vi "HandshakeResponse.vi"(8 "error in (no error)":errorcluster, 10 "Sec-WebSocket-Key":string, 11 "WebSocket In":refnum<class "WebSocket.lvclass">) -> (0 "error out":errorcluster, 2 "Response Headers":string, 3 "WebSocket out":refnum<class "WebSocket.lvclass">)   [LabVIEW 2021, in "WebSockets.lvlib" / "WebSocket.lvclass"]
doc: "Creates the HTTP handshaking response.\nWebSockets 2.0.1.40\nSam Sharp - MediaMongrels Ltd\nCopyright (c) 2019, MediaMongrels Ltd"
uses:
  WebSocket.lvclass
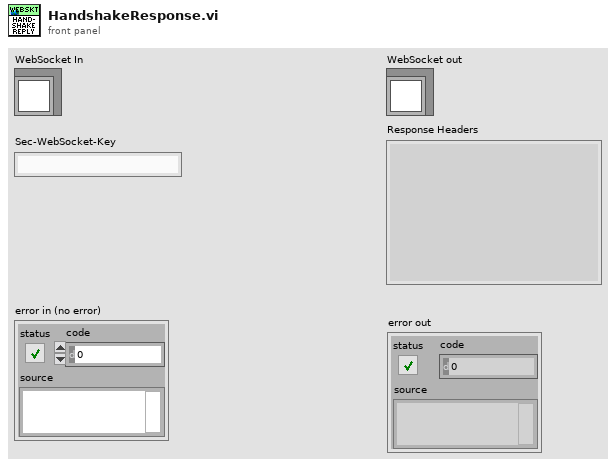
[diagram p1: front panel]
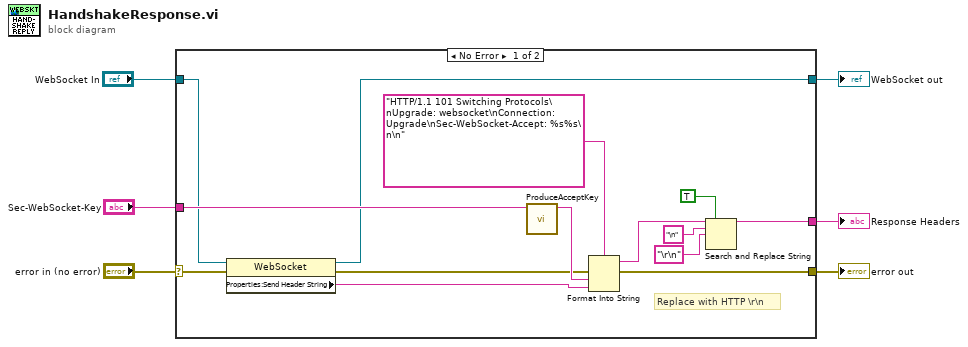
[diagram p0: block diagram]
diagram:
  n1 = case shown="No Error" "error in (no error)" {
    selector: "error in (no error)" -> [w17 w22]
    tunnel: "Sec-WebSocket-Key" -> [w20 _]
    tunnel: [w12 _] -> w5
    tunnel: [w18 w22] -> w3
    tunnel: "WebSocket In" -> [w10 w21]
    tunnel: [w7 w21] -> w1
    frame No Error {
      # "Replace with HTTP \\r\\n"
      n2 = property class="WebSocket"(reference=w10, error in=w17) -> (reference out=w7:refnum<class "WebSocket.lvclass">, error out=w11:errorcluster, "Properties:Send Header String"=w9:string)
      n3 = call "ProduceAcceptKey.vi"("Sec-WebSocket-Key"=w20) -> ("Sec-WebSocket-Accept"=w19:string)  [unwired: 10 in]
      n4 = Format Into String(format string="HTTP/1.1 101 Switching Protocols\nUpgrade: websocket\nConnection: Upgrade\nSec-WebSocket-Accept: %s%s\n\n", error in=w11, w19, w9) -> (resulting string=w13:string, error out=w18:errorcluster)  [unwired: 1 in]
      n5 = Search and Replace String(replace all?=TRUE ("replace all? (F)"), input string=w13, search string="\n" ("search string/char (-)"), replace string="\r\n" ("search string/char (-)")) -> (result string=w12:string)  [unwired: 4 in, 3 out]
    }
    frame Error {
    }
  }
  "Response Headers" <- w5
  "error out" <- w3
  "WebSocket out" <- w1
